vi "ReadSpeed.vi"(8 "error in":errorcluster, 10 "milliseconds to wait":u32=50, 11 "VISA resource name":refnum<visa-resource-name>) -> (0 "error out":errorcluster, 2 "Speed":dbl, 3 "VISA resource name out":refnum<visa-resource-name>)   [LabVIEW 2019, in "Mark 10 TSTM-DC.lvlib"]
uses:
  Mark 10 TSTM-DC.lvlib
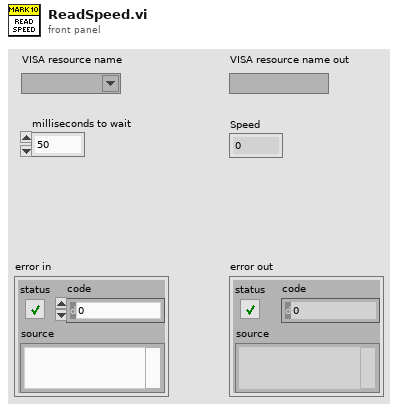
[diagram p1: front panel]
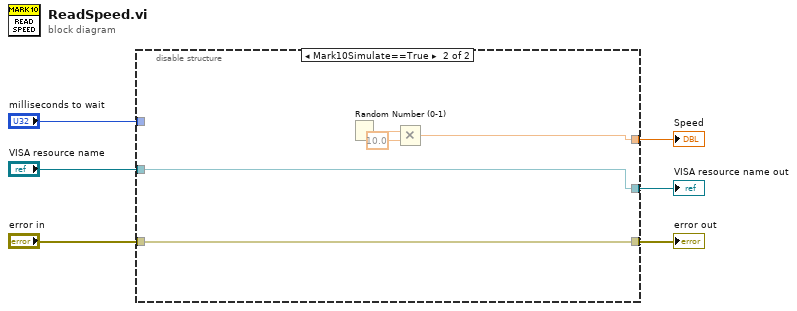
[diagram p0: block diagram]
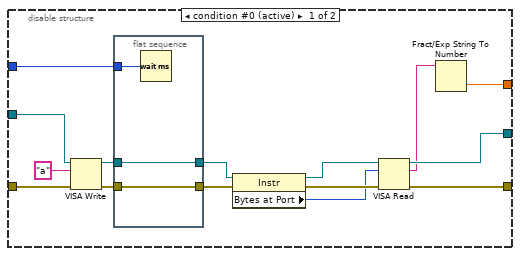
[diagram p2: hidden frame]
diagram:
  n1 = disable-structure shown="Mark10Simulate==True" {
    disable-tunnel: [w20 w29] -> w6
    disable-tunnel: "VISA resource name" -> [w19 w29]
    disable-tunnel: "error in" -> [w18 w28]
    disable-tunnel: [w17 w28] -> w3
    disable-tunnel: [w16 w25] -> w2
    disable-tunnel: "milliseconds to wait" -> [w7 _]
    frame condition #0 (active) {
      n2 = VISA Write(VISA resource name=w19, write buffer="a" ("String to Write"), error in (no error)=w18) -> (VISA resource name out=w12:refnum<visa-resource-name>, error out=w11:errorcluster)  [unwired: 1 out]
      n3 = flat-sequence {
        tunnel: [w24] -> w13
        tunnel: w12 -> [w24]
        tunnel: w11 -> [w23]
        tunnel: [w23] -> w10
        tunnel: w7 -> [w22]
        frame #0 {
          n4 = Wait (ms)(milliseconds to wait=w22) -> ()  [unwired: 1 out]
        }
      }
      n5 = property class="Instr"(reference=w13, error in=w10) -> (reference out=w14:refnum<visa-resource-name>, error out=w15:errorcluster, "Bytes at Port"=w8:u32)
      n6 = VISA Read(VISA resource name=w14, byte count=w8, error in (no error)=w15) -> (VISA resource name out=w20:refnum<visa-resource-name>, read buffer=w9:string, error out=w17:errorcluster)  [unwired: 1 out]
      n7 = Fract/Exp String To Number(string=w9) -> (number=w16:dbl)  [unwired: 3 in, 1 out]
    }
    frame condition #1 {
      n8 = Random Number (0-1)() -> (number: 0 to 1=w27:dbl)
      n9 = Multiply(x=w27, y=10.0) -> (x*y=w25:dbl)
    }
  }
  "error out" <- w3
  "VISA resource name out" <- w6
  "Speed" <- w2
